vi "_GetSourceType.vi"(6 "error in (no error)":errorcluster, 9 "node in":refnum<k20>) -> (0 "ESI2":string, 1 "ESI1":string, 2 "APCI2":string, 3 "APCI1":string, 4 "HasESI2":bool, 5 "HasESI1":bool)   [LabVIEW 2015]
uses:
  <vilib>/xml/Close Reference(Node).vi
  <vilib>/xml/NI_XML.lvlib
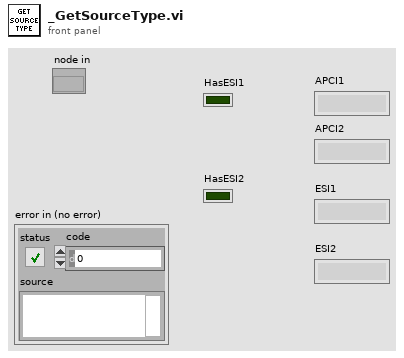
[diagram p1: front panel]
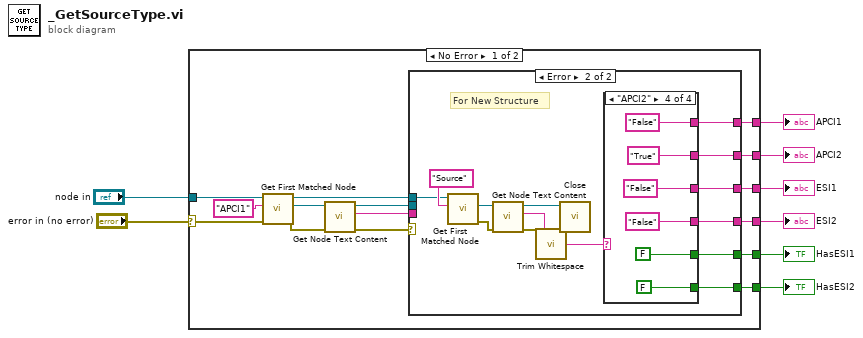
[diagram p0: block diagram]
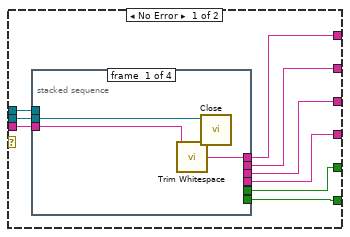
[diagram p2: hidden frame]
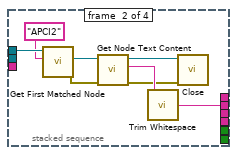
[diagram p3: hidden frame]
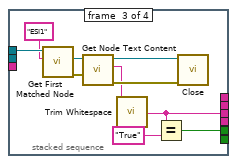
[diagram p4: hidden frame]
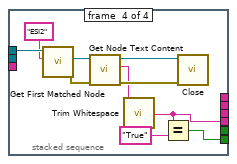
[diagram p5: hidden frame]
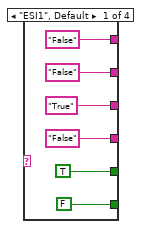
[diagram p6: hidden frame]
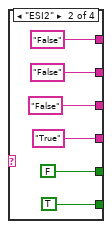
[diagram p7: hidden frame]
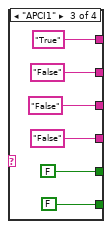
[diagram p8: hidden frame]
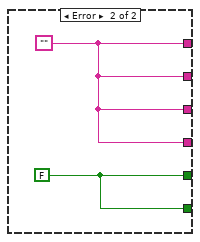
[diagram p9: hidden frame]
diagram:
  n1 = case shown="No Error" "error in (no error)" {
    selector: "error in (no error)" -> [w10 _]
    tunnel: [w21 w103] -> w7
    tunnel: [w20 w103] -> w6
    tunnel: [w19 w103] -> w5
    tunnel: [w18 w103] -> w4
    tunnel: [w17 w102] -> w3
    tunnel: [w16 w102] -> w2
    tunnel: "node in" -> [w9 _]
    frame No Error {
      n2 = call <vilib>:"Get First Matched Node.vi"("error in (no error)"=w10, "XPath expression"="APCI1", "node in"=w9) -> ("error out"=w14:errorcluster, "node result"=w15:refnum<k20>, "node out"=w22:refnum<k20>)  [unwired: 6 in]
      n3 = call <vilib>:"Get Node Text Content.vi"("error in (no error)"=w14, "node in"=w15) -> ("error out"=w13:errorcluster, "node text"=w11:string, "node out"=w12:refnum<k20>)  [unwired: 7 in]
      n4 = case shown="Error" w13 {
        tunnel: w22 -> [w32 w76]
        tunnel: [w31 w69] -> w21
        tunnel: [w30 w68] -> w20
        tunnel: [w29 w67] -> w19
        tunnel: [w28 w66] -> w18
        tunnel: [w27 w65] -> w17
        tunnel: [w26 w64] -> w16
        tunnel: w12 -> [w25 _]
        tunnel: w11 -> [w24 _]
        frame No Error {
          n5 = stacked-sequence {
            tunnel: w32 -> [_ w43 w53 w63]
            tunnel: [w35 _ _ _] -> w31
            tunnel: [_ w36 _ _] -> w30
            tunnel: [_ _ w46 _] -> w29
            tunnel: [_ _ _ w55] -> w28
            tunnel: [_ _ _ w54] -> w26
            tunnel: [_ _ w44 _] -> w27
            tunnel: w25 -> [w34 _ _ _]
            tunnel: w24 -> [w33 _ _ _]
            frame #0 {
              n6 = call <vilib>:"Trim Whitespace.vi"("string"=w33) -> ("trimmed string"=w35:string)  [unwired: 1 in]
              n7 = call-poly <vilib>:"Close.vi"("node"=w34) -> ()  [unwired: 8 in, 1 out]
            }
            frame #1 {
              n8 = call <vilib>:"Get First Matched Node.vi"("XPath expression"="APCI2", "node in"=w43) -> ("error out"=w37:errorcluster, "node result"=w41:refnum<k20>)  [unwired: 7 in, 1 out]
              n9 = call <vilib>:"Get Node Text Content.vi"("error in (no error)"=w37, "node in"=w41) -> ("error out"=w38:errorcluster, "node text"=w40:string, "node out"=w39:refnum<k20>)  [unwired: 7 in]
              n10 = call <vilib>:"Trim Whitespace.vi"("string"=w40) -> ("trimmed string"=w36:string)  [unwired: 1 in]
              n11 = call-poly <vilib>:"Close.vi"("error in (no error)"=w38, "node"=w39) -> ()  [unwired: 7 in, 1 out]
            }
            frame #2 {
              n12 = call <vilib>:"Get First Matched Node.vi"("XPath expression"="ESI1", "node in"=w53) -> ("error out"=w50:errorcluster, "node result"=w51:refnum<k20>)  [unwired: 7 in, 1 out]
              n13 = call <vilib>:"Get Node Text Content.vi"("error in (no error)"=w50, "node in"=w51) -> ("error out"=w49:errorcluster, "node text"=w47:string, "node out"=w48:refnum<k20>)  [unwired: 7 in]
              n14 = call <vilib>:"Trim Whitespace.vi"("string"=w47) -> ("trimmed string"=w46:string)  [unwired: 1 in]
              n15 = Equal?(x=w46, y="True") -> (x = y?=w44:bool)
              n16 = call-poly <vilib>:"Close.vi"("error in (no error)"=w49, "node"=w48) -> ()  [unwired: 7 in, 1 out]
            }
            frame #3 {
              n17 = call <vilib>:"Get First Matched Node.vi"("XPath expression"="ESI2", "node in"=w63) -> ("error out"=w60:errorcluster, "node result"=w61:refnum<k20>)  [unwired: 7 in, 1 out]
              n18 = call <vilib>:"Get Node Text Content.vi"("error in (no error)"=w60, "node in"=w61) -> ("error out"=w58:errorcluster, "node text"=w56:string, "node out"=w59:refnum<k20>)  [unwired: 7 in]
              n19 = call <vilib>:"Trim Whitespace.vi"("string"=w56) -> ("trimmed string"=w55:string)  [unwired: 1 in]
              n20 = Equal?(x=w55, y="True") -> (x = y?=w54:bool)
              n21 = call-poly <vilib>:"Close.vi"("error in (no error)"=w58, "node"=w59) -> ()  [unwired: 7 in, 1 out]
            }
          }
        }
        frame Error {
          # "For New Structure"
          n22 = call <vilib>:"Get First Matched Node.vi"("XPath expression"="Source", "node in"=w76) -> ("error out"=w71:errorcluster, "node result"=w72:refnum<k20>)  [unwired: 7 in, 1 out]
          n23 = call <vilib>:"Get Node Text Content.vi"("error in (no error)"=w71, "node in"=w72) -> ("error out"=w74:errorcluster, "node text"=w73:string, "node out"=w75:refnum<k20>)  [unwired: 7 in]
          n24 = call <vilib>:"Trim Whitespace.vi"("string"=w73) -> ("trimmed string"=w70:string)  [unwired: 1 in]
          n25 = call-poly <vilib>:"Close.vi"("error in (no error)"=w74, "node"=w75) -> ()  [unwired: 7 in, 1 out]
          n26 = case shown="\"APCI2\"" w70 {
            tunnel: ["False" ("y") "False" ("y") "True" ("y") "False" ("y")] -> w69
            tunnel: ["False" ("y") "False" ("y") "False" ("y") "True" ("y")] -> w68
            tunnel: ["True" ("y") "False" ("y") "False" ("y") "False" ("y")] -> w67
            tunnel: ["False" ("y") "True" ("y") "False" ("y") "False" ("y")] -> w66
            tunnel: [TRUE FALSE FALSE FALSE] -> w65
            tunnel: [FALSE TRUE FALSE FALSE] -> w64
            frame "ESI1", Default {
            }
            frame "ESI2" {
            }
            frame "APCI1" {
            }
            frame "APCI2" {
            }
          }
        }
      }
    }
    frame Error {
      w102 = FALSE
      w103 = ""
    }
  }
  "ESI1" <- w5
  "ESI2" <- w4
  "APCI1" <- w7
  "APCI2" <- w6
  "HasESI1" <- w3
  "HasESI2" <- w2
